vi "tree_state_interface.vi"   [LabVIEW 2020]
uses:
  state/state.lvclass
  1ccf8ff9-ab9b-412d-8cf6-df7dccfd1160.vi
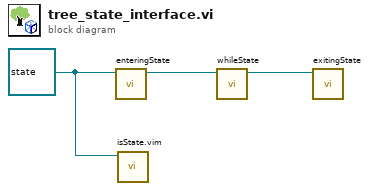
[diagram p0: block diagram]
diagram:
  w1 = refnum<class "state.lvclass"> refnum ("eos.lvlib:state.lvclass")
  n1 = call-dynamic "enteringState.vi"("state in"=w1) -> ("state out"=w2:refnum<class "state.lvclass">)  [unwired: 9 in, 1 out]
  n2 = call "isState.vim"("Object"=w1) -> ()  [unwired: 9 in, 2 out]
  n3 = call-dynamic "whileState.vi"("state in"=w2) -> ("state out"=w3:refnum<class "state.lvclass">)  [unwired: 9 in, 1 out]
  n4 = call-dynamic "exitingState.vi"("state in"=w3) -> ()  [unwired: 9 in, 2 out]
